vi "FL_Reshape_data_back_for_saving_(strings).vi"(1 "Read frame size":u32=8, 2 "DEC string input":string[](array[string])) -> (0 "DEC string output":string[][](array[string]))   [LabVIEW 2016]
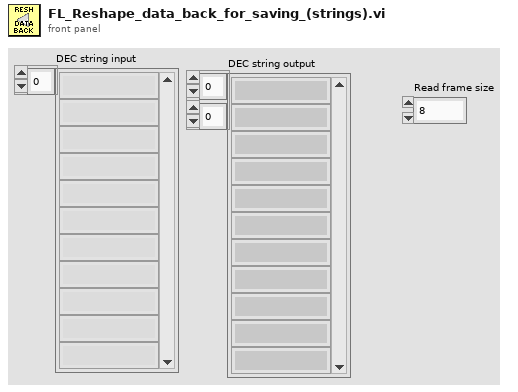
[diagram p1: front panel]
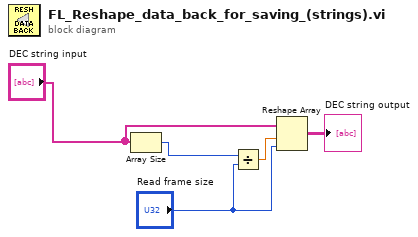
[diagram p0: block diagram]
diagram:
  n1 = Array Size(array="DEC string input") -> (size(s)=w3:i32)
  n2 = Divide(x=w3, y="Read frame size") -> (x/y=w4:dbl)
  n3 = Reshape Array("DEC string input", w4, "Read frame size") -> (→"DEC string output":string[][])
